vi "DetectActive Channels.vi"(8 "error in (no error)":errorcluster, 11 "resourcename in":string) -> (0 "error out":errorcluster, 2 "Array":u16[](array[numeric]), 3 "resourcename out":string)   [LabVIEW 2013, in "TektronixDPOSimple.lvclass"]
uses:
  TektronixDPOSimple.lvclass
  Tektronix DPO MSO 2000 4000 Series.lvlib
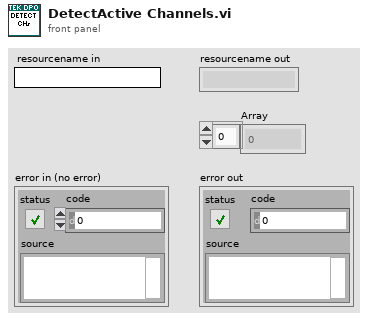
[diagram p1: front panel]
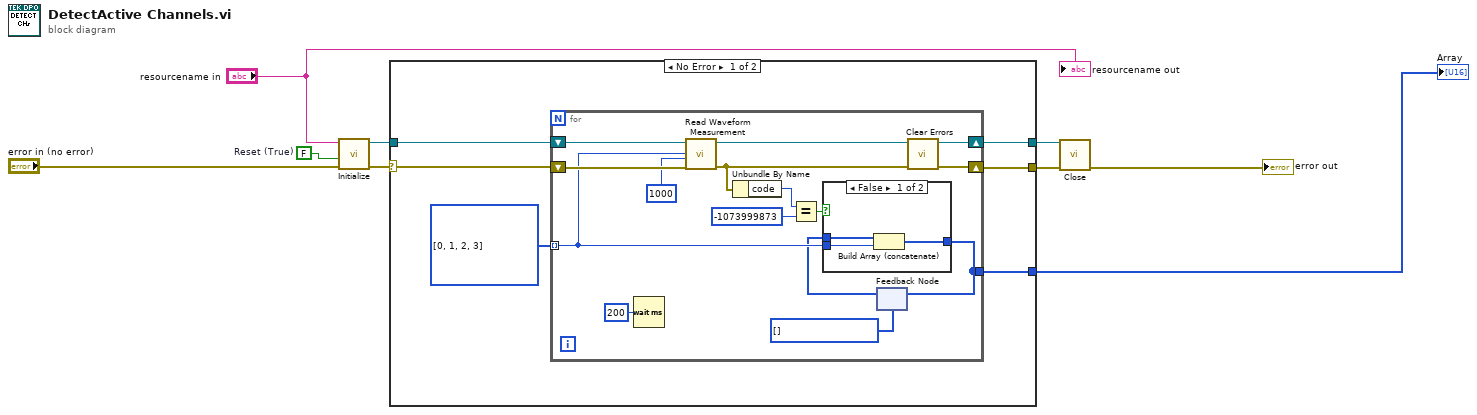
[diagram p0: block diagram]
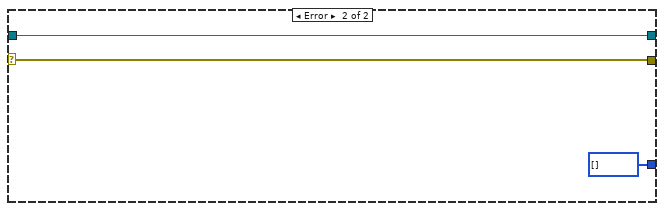
[diagram p3: hidden frame]
diagram:
  w7 = FALSE  # Reset (True)
  n1 = call "Initialize.vi"("error in (no error)"="error in (no error)", "Reset (True)"=w7, "VISA resource name"="resourcename in") -> ("error out"=w9:errorcluster, "VISA resource name out"=w2:refnum<visa-resource-name>)  [unwired: 7 in]
  n2 = case shown="No Error" w9 {
    selector: w9 -> [w10 w36]
    tunnel: w2 -> [w15 w35]
    tunnel: [w14 w35] -> w4
    tunnel: [w13 w36] -> w5
    tunnel: [w11 u16[] []] -> w8
    frame No Error {
      w12 = u16[] [0, 1, 2, 3] items=["Channel 1", "Channel 2", "Channel 3", "Channel 4", "Math", "Reference 1", "Reference 2", "Reference 3", "Reference 4", "D0", "D1", "D2", "D3", "D4", "D5", "D6", "D7", "D8", "D9", "D10", "D11", "D12", "D13", "D14", "D15", "Amplitude", "Frequency", "Phase", "Normal", "Average", "Maximum Peak Hold", "Minimum Peak Hold"]
      n3 = for {
        tunnel: w12 -> [w19] mode=indexing
        shift-right: [w26] -> w14
        shift-left: w15 -> [w27]
        shift-right: [w28] -> w13
        shift-left: w10 -> [w25]
        tunnel: [w16] -> w11
        w17 = u16[] [] items=["Channel 1", "Channel 2", "Channel 3", "Channel 4", "Math", "Reference 1", "Reference 2", "Reference 3", "Reference 4", "D0", "D1", "D2", "D3", "D4", "D5", "D6", "D7", "D8", "D9", "D10", "D11", "D12", "D13", "D14", "D15", "Amplitude", "Frequency", "Phase", "Normal", "Average", "Maximum Peak Hold", "Minimum Peak Hold"]
        n4 = Wait (ms)(milliseconds to wait=u32 200) -> ()  [unwired: 1 out]
        n5 = call "Read Waveform Measurement.vi"("error in (no error)"=w25, "Maximum Time (10000ms)"=u32 1000, "Channel (0: Channel 1)"=w19, "VISA resource name"=w27) -> ("error out"=w23:errorcluster, "VISA resource name out"=w26:refnum<visa-resource-name>)  [unwired: 5 in, 1 out]
        n6 = Unbundle By Name(w23) -> ("code"=w22:i32)
        n7 = Equal?(x=w22, y=-1073999873) -> (x = y?=w20:bool)
        n8 = feedback #1(w17) -> (w18:u16[])
        n9 = case shown="False" w20 {
          tunnel: w19 -> [w31 _]
          tunnel: w18 -> [w32 w33]
          tunnel: [w30 w33] -> w16
          frame False {
            n10 = Build Array (concatenate)(w32, w31) -> (w30:u16[])
          }
          frame True {
          }
        }
        n11 = feedback-in #1(w16) -> ()
        n12 = call "Clear Errors.vi"("error in (no error)"=w23) -> ("error out"=w28:errorcluster)  [unwired: 6 in]
      }
    }
    frame Error {
    }
  }
  "Array" <- w8
  n13 = call "Close.vi"("error in (no error)"=w5, "VISA resource name"=w4) -> ("error out"=→"error out":errorcluster)  [unwired: 9 in]
  "resourcename out" <- "resourcename in"
